vi "Wave1D_Init Data_Delta.vi"(11 "Domain":T1={"t"={"initial t"=0.0, "final t"=1.0, "# of t-points"=11}, "x"={"start x"=0.0, "end x"=1.0, "# of x-points"=11}}) -> (2 "delta x":dbl, 3 "delta t":dbl)   [LabVIEW 2017, in "NI_PDE.lvlib"]
uses:
  <vilib>/gmath/NI_PDE.lvlib
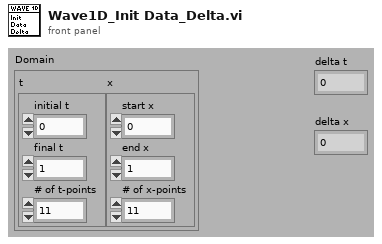
[diagram p1: front panel]
types:
  T1 = cluster{"t":cluster{"initial t":dbl, "final t":dbl, "# of t-points":i32}, "x":cluster{"start x":dbl, "end x":dbl, "# of x-points":i32}}
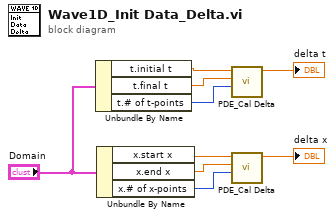
[diagram p0: block diagram]
diagram:
  n1 = Unbundle By Name("Domain") -> ("t.initial t"=w9:dbl, "t.final t"=w8:dbl, "t.# of t-points"=w7:i32)
  n2 = Unbundle By Name("Domain") -> ("x.start x"=w4:dbl, "x.end x"=w5:dbl, "x.# of x-points"=w6:i32)
  n3 = call <vilib>:"PDE_Cal Delta.vi"("# of points"=w7, "end"=w8, "start"=w9) -> ("delta"=→"delta t":dbl)  [unwired: 8 out]
  n4 = call <vilib>:"PDE_Cal Delta.vi"("# of points"=w6, "end"=w5, "start"=w4) -> ("delta"=→"delta x":dbl)  [unwired: 8 out]
